vi "Close.vi"(8 "error in (no error)":errorcluster, 11 "CIPC Reference":u64) -> (0 "error out":errorcluster)   [LabVIEW 2021, in "CIF_NI_CIPC.lvlib"]
doc: "Close the reference to the buffer without destroying the buffer."
uses:
  CIF_NI_CIPC.lvlib
  SubVIs/Check Error.vi
  SubVIs/Get dll Path.vi
  <vilib>/Utility/error.llb/Trim Whitespace.vi
  <vilib>/Utility/error.llb/Error Cluster From Error Code.vi
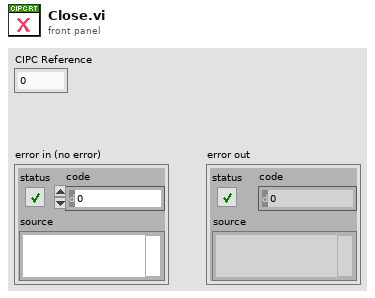
[diagram p1: front panel]
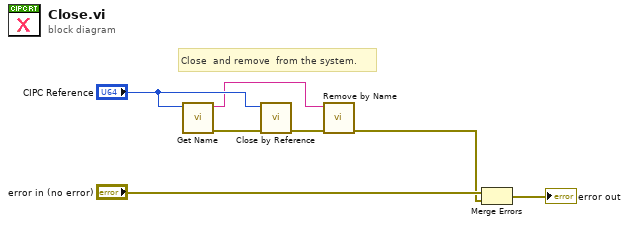
[diagram p0: block diagram]
diagram:
  # "Close  and remove  from the system."
  n1 = call "Get Name.vi"("CIPC Reference"="CIPC Reference") -> ("error out"=w5:errorcluster, "Name"=w3:string)  [unwired: 9 in]
  n2 = call "Close by Reference.vi"("error in (no error)"=w5, "CIPC Reference"="CIPC Reference") -> ("error out"=w4:errorcluster)  [unwired: 9 in]
  n3 = call "Remove by Name.vi"("error in (no error)"=w4, "buffer_name"=w3) -> ("error out"=w1:errorcluster)  [unwired: 9 in]
  n4 = Merge Errors("error in (no error)", w1) -> (→"error out":errorcluster)
